vi "RS Bistable.vi"(8 "error in":errorcluster, 10 "reset":bool, 11 "set":bool) -> (0 "error out":errorcluster, 3 "output":bool)   [LabVIEW 2017, in "NI_FunctionBlock Libraries.lvlib"]
uses:
  <vilib>/functionblocks/NI_FunctionBlock Libraries.lvlib
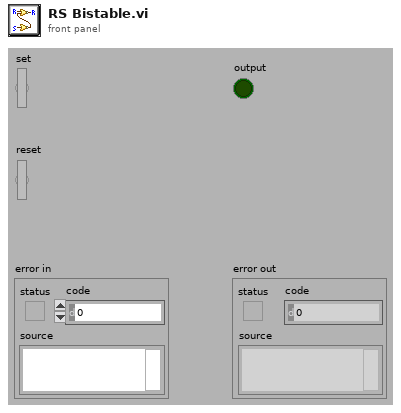
[diagram p1: front panel]
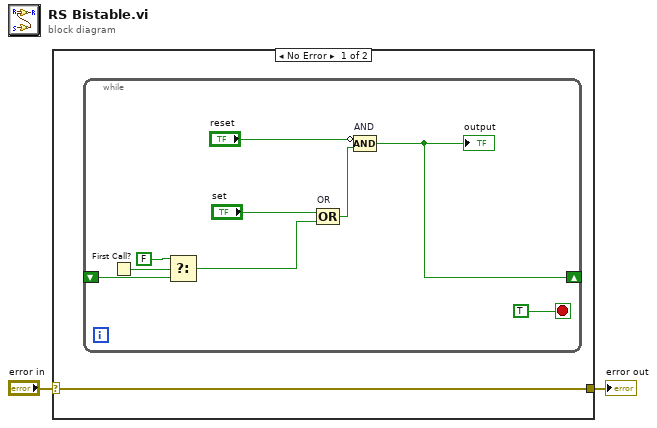
[diagram p0: block diagram]
diagram:
  n1 = case shown="No Error" "error in" {
    selector: "error in" -> [w3 w13]
    tunnel: [w3 w13] -> w1
    frame No Error {
      n2 = while {
        shift-right: [w6] -> _
        shift-left: _ -> [w5]
        stop <- TRUE stop-if-true
        n3 = First Call?() -> (First Call?: T/F=w12:bool)
        n4 = Select(t=FALSE, s=w12, f=w5) -> (s? t:f=w10:bool)
        n5 = Compound Arithmetic op=OR "OR"("set", w10) -> (w9:bool)
        n6 = Compound Arithmetic op=AND "AND"(invert "reset", w9) -> (w6:bool)
        "output" <- w6
      }
    }
    frame Error {
    }
  }
  "error out" <- w1
